vi "Process Producto.vi"(8 "error in (no error)":errorcluster, 10 "Producto":enum16{"Coca", "Fanta", "Manzanita", "Ciel"}(ring), 11 "MXN Actor in":refnum<class "MXN Actor.lvclass">) -> (0 "error out":errorcluster, 3 "MXN Actor out":refnum<class "MXN Actor.lvclass">)   [LabVIEW 2020]
uses:
  MXN Actor.lvclass
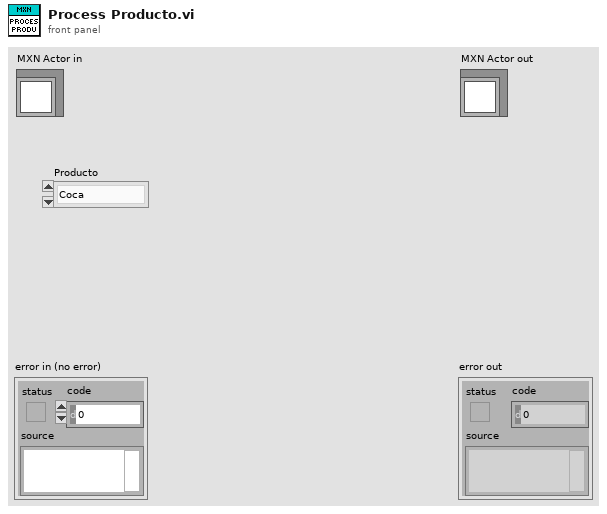
[diagram p1: front panel]
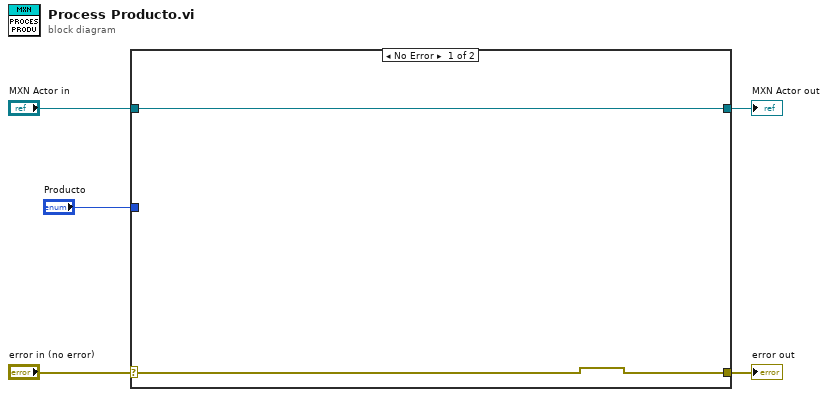
[diagram p0: block diagram]
diagram:
  n1 = case shown="No Error" "error in (no error)" {
    selector: "error in (no error)" -> [w6 w9]
    tunnel: [w6 w9] -> w4
    tunnel: [w7 w8] -> w2
    tunnel: "MXN Actor in" -> [w7 w8]
    tunnel: "Producto" -> [_ _]
    frame No Error {
    }
    frame Error {
    }
  }
  "error out" <- w4
  "MXN Actor out" <- w2
